vi "trio_move.vi"(6 "Axis enable":bool[](array[boolean])=[TRUE, TRUE, TRUE, TRUE], 7 "Timeout (ms)":u32=10000, 8 "error in":errorcluster, 9 "Axis positions":dbl[](array[numeric])=[0.0, 0.0, 0.0, 0.0], 10 "Absolute":bool=TRUE, 11 "Trio handle":refnum<k7>) -> (0 "error out":errorcluster)   [LabVIEW 2024]
uses:
  <instrlib>/Trio Motion/Trio Motion Library.lvlib
panel:
  out "Moving axes":bool[](array[boolean])
  in  "Poll delay (ms)":u32=50
  # "How long to wait for motion to complete."
  # "The purposes of axis enable is to allow a subset of axes to be driven in absolute position mode without changing (or knowing) the positions of the other axes.   Being disabled just means that we don't want to move that axis, not that we want it powered down."
  # "How long to wait when polling for motion completion"
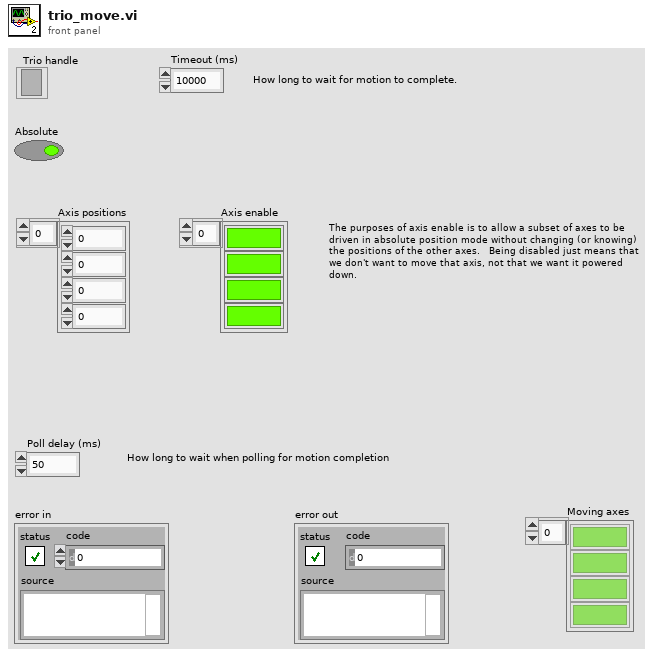
[diagram p1: front panel]
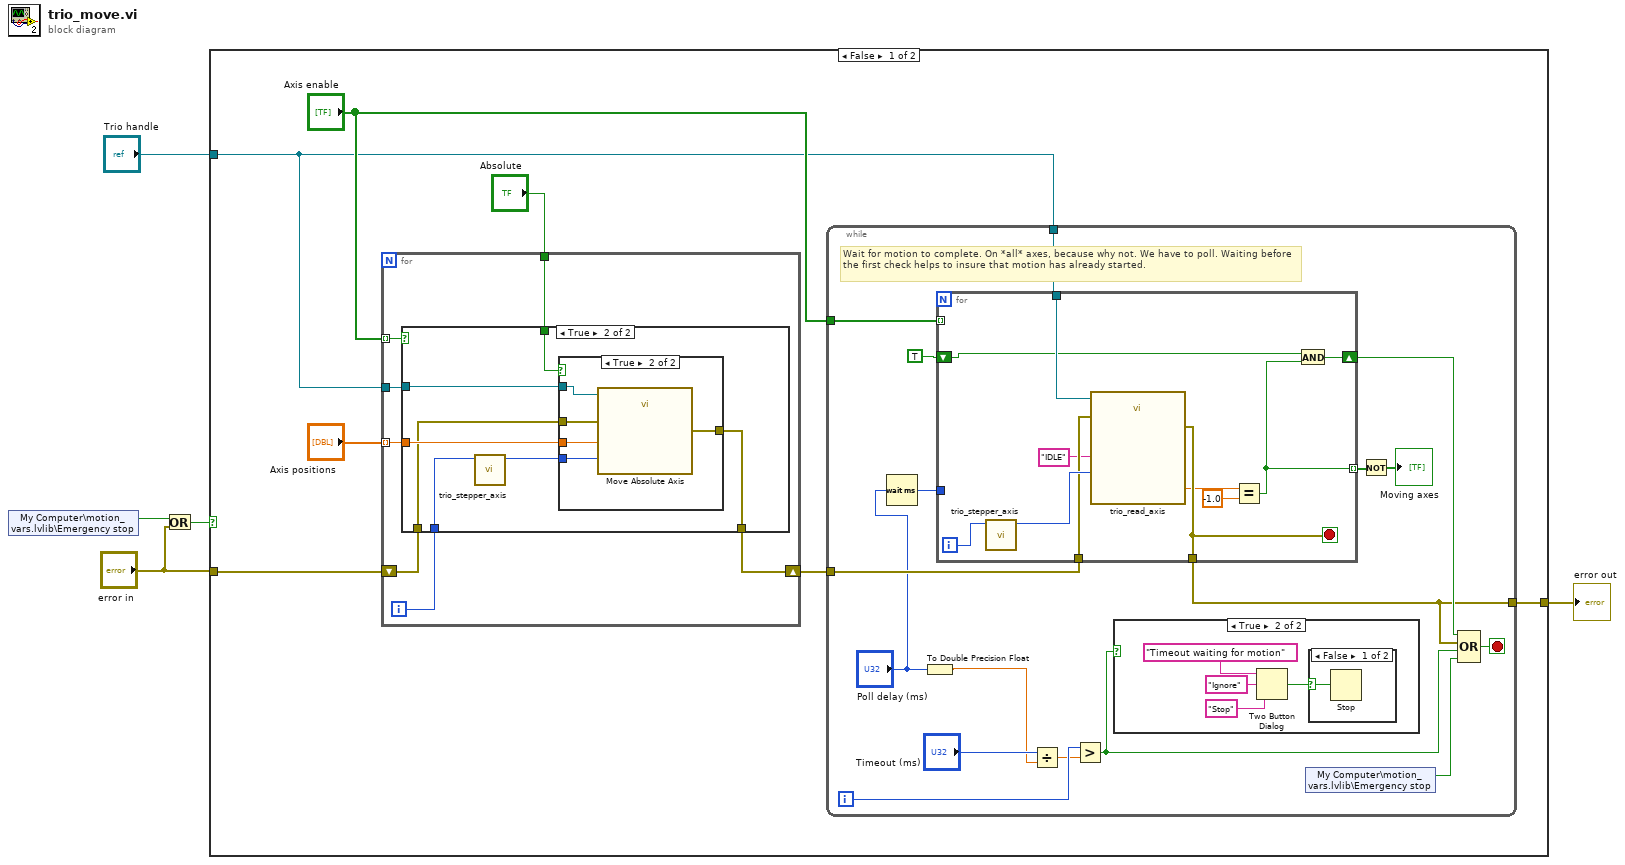
[diagram p0: block diagram]
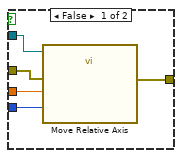
[diagram p5: hidden frame]
diagram:
  n1 = shared-variable "My Computer\\motion_vars.lvlib\\Emergency stop"() -> (w4:bool)  [unwired: 1 in, 1 out]
  n2 = Or(x=w4, y="error in") -> (x .or. y?=w2:bool)
  n3 = case shown="False" w2 {
    tunnel: "error in" -> [w11 w71]
    tunnel: [w6 w71] -> w5
    tunnel: "Trio handle" -> [w7 _]
    frame False {
      n4 = for {
        tunnel: "Axis enable" -> [w51] mode=indexing
        tunnel: "Axis positions" -> [w50] mode=indexing
        shift-right: [w49] -> w8
        shift-left: w11 -> [w52]
        tunnel: "Absolute" -> [w47]
        tunnel: w7 -> [w46]
        i -> [w48]
        n5 = case shown="True" w51 {
          tunnel: w52 -> [w53 w56]
          tunnel: w48 -> [_ w54]
          tunnel: w50 -> [_ w59]
          tunnel: [w53 w57] -> w49
          tunnel: w47 -> [_ w60]
          tunnel: w46 -> [_ w58]
          frame False {
          }
          frame True {
            n6 = call "trio_stepper_axis.vi"("Encoder axis"=w54) -> ("Stepper axis"=w55:i32)  [unwired: 10 in]
            n7 = case shown="True" w60 {
              tunnel: w59 -> [w65 w67]
              tunnel: w56 -> [w64 w68]
              tunnel: w55 -> [w63 w66]
              tunnel: w58 -> [w62 w69]
              tunnel: [w61 w70] -> w57
              frame False {
                n8 = call <instrlib>:"Move Relative Axis.vi"("error in (no error)"=w64, "Distance"=w65, "Axis (0)"=w63, "reference in"=w62) -> ("error out"=w61:errorcluster)  [unwired: 5 in, 2 out]
              }
              frame True {
                n9 = call <instrlib>:"Move Absolute Axis.vi"("error in (no error)"=w68, "Position"=w67, "Axis (0)"=w66, "reference in"=w69) -> ("error out"=w70:errorcluster)  [unwired: 5 in, 2 out]
              }
            }
          }
        }
      }
      n10 = while {
        tunnel: "Axis enable" -> [w29]
        tunnel: w8 -> [w28]
        tunnel: w7 -> [w27]
        tunnel: [w23] -> w6
        i -> [w19]
        stop <- w25 stop-if-true
        # "Wait for motion to complete. On *all* axes, because why not. We have to poll. Waiting before the first check helps to insure that motion has already started."
        n11 = Wait (ms)(milliseconds to wait="Poll delay (ms)") -> (millisecond timer value=w22:u32)
        n12 = To Double Precision Float(number="Poll delay (ms)") -> (double precision float=w13:dbl)
        n13 = for {
          tunnel: w29 -> [_] mode=indexing
          tunnel: w28 -> [w43]
          tunnel: w27 -> [w42]
          tunnel: [w40] -> w23
          shift-right: [w37] -> w24
          shift-left: TRUE -> [w36]
          tunnel: w22 -> [_]
          tunnel: [w35] -> w15 mode=indexing
          i -> [w45]
          stop <- w40 stop-if-true
          n14 = call "trio_stepper_axis.vi"("Encoder axis"=w45) -> ("Stepper axis"=w44:i32)  [unwired: 10 in]
          n15 = call "trio_read_axis.vi"("Axis"=w44, "error in (no error)"=w43, "Variable"="IDLE", "reference in"=w42) -> ("error out"=w40:errorcluster, "Value"=w39:dbl)  [unwired: 5 in, 1 out]
          n16 = Equal?(x=w39, y=-1.0) -> (x = y?=w35:bool)
          n17 = And(x=w36, y=w35) -> (x .and. y?=w37:bool)
        }
        n18 = Divide(x="Timeout (ms)", y=w13) -> (x/y=w18:dbl)
        n19 = Greater?(x=w19, y=w18) -> (0:w16:bool)
        n20 = case shown="True" w16 {
          frame False {
          }
          frame True {
            n21 = Two Button Dialog(message="Timeout waiting for motion", 1:"Stop" ("F button name (\"Cancel\")"), 2:"Ignore" ("T button name (\"OK\")")) -> (T button?=w30:bool)
            n22 = case shown="False" w30 {
              selector: w30 -> [w34 _]
              frame False {
                n23 = Stop(stop? (T)=w34) -> ()
              }
              frame True {
              }
            }
          }
        }
        n24 = shared-variable "My Computer\\motion_vars.lvlib\\Emergency stop"() -> (w17:bool)  [unwired: 1 in, 1 out]
        n25 = Not(x=w15) -> (.not. x?=→"Moving axes":bool[])
        n26 = Compound Arithmetic op=OR(w24, w23, w16, w17) -> (w25:bool)
      }
    }
    frame True {
    }
  }
  "error out" <- w5
